vi "Read XML_Convert Rx XML SDI Element to SDIVAlue and SDI_Enabled.vi"(11 "SDI":i32) -> (1 "SDI_Enabled":bool, 3 "SDIValue":u8)   [LabVIEW 2016]
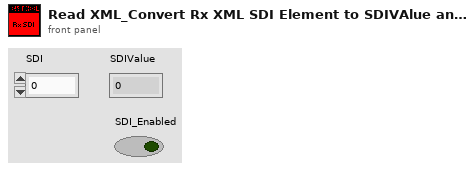
[diagram p1: front panel]
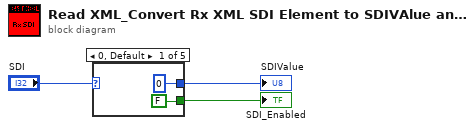
[diagram p0: block diagram]
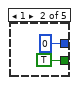
[diagram p2: hidden frame]
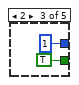
[diagram p3: hidden frame]
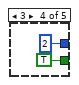
[diagram p4: hidden frame]
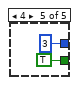
[diagram p5: hidden frame]
diagram:
  n1 = case shown="0, Default" "SDI" {
    tunnel: [FALSE TRUE TRUE TRUE TRUE] -> w2
    tunnel: [u8 0 ("SDIValue") u8 0 ("SDIValue") u8 1 ("SDIValue") u8 2 ("SDIValue") u8 3 ("SDIValue")] -> w3
    frame 0, Default {
    }
    frame 1 {
    }
    frame 2 {
    }
    frame 3 {
    }
    frame 4 {
    }
  }
  "SDIValue" <- w3
  "SDI_Enabled" <- w2
